vi "Pressure_cuff_3_tyler edit.vi"() -> ()   [LabVIEW 2016]
uses:
  <vilib>/Utility/miscctls.llb/LVBoundsTypeDef.ctl
  <vilib>/Instr/_visa.llb/VISA Configure Serial Port (Instr).vi
  <vilib>/Utility/file.llb/Write To Spreadsheet File (DBL).vi
  <vilib>/ptbypt/NI_PtbyPt.lvlib
panel:
  in  "?":enum32{"Serial Commands", "Operation"}(tab)
  in  "?":string="Instructions:\n\n1) Adjust Serial Commands appropriately using the \"Serial Commands\" tab and following the associated instructions.\n\nNote: There are two modes built into this system. The most basic mode is the \"Manual\" mode in which the continually defines the desired pressure throughout the experiment. The second mode is the \"Automatic\" mode in which the user can obtain a stair-step response by increasing/decreasing the pressure by user-defined increments of pressure every user-defined length of time.\n\n*When the \"Sync Auto/Manual\" indicator is illuminated, the program will maintain the same pressure when the user switches back and forth between the Manual and Automatic modes. This is the default setting."
  in  "Set Pump Mode":string="MOD PMP\r\n"
  in  "Set Diameter":string="11.001"
  in  "Set Direction to Refill":string="DIR REF\r\n"
  in  "Run1":string="RUN\r\n"
  in  "Stop":string="STP\r\n"
  in  "Set Fast Infusion Rate":string="1.0600"
  in  "Run":string="RUN\r\n"
  in  "Run4":string="RUN\r\n"
  in  "Set Direction to Infuse 2":string="DIR INF\r\n"
  in  "Run2":string="RUN\r\n"
  in  "Set Slow Infusion Rate":string="250.02"
  in  "Set Direction to Refill 2":string="DIR REF\r\n"
  in  "Run3":string="RUN\r\n"
  in  "Set Slow to Refill Rate":string="250.05"
  in  "Set Fast Refill Rate":string="1.0003"
  in  "Set Direction to Infuse":string="DIR INF\r\n"
  in  "D1":string="DIA "
  in  "D3":string="\r\n"
  in  "Set FRR":string="RFR "
  in  "Set FRR1":string=" MM\r\n"
  in  "Set FIR":string="RAT "
  in  "Set FIR1":string=" MM\r\n"
  in  "Set SIR":string="RAT "
  in  "Set SIR1":string=" UM\r\n"
  in  "Set SRR":string="RFR "
  in  "Set SRR1":string=" UM\r\n"
  in  "Set Initial Refill Rt":string="RFR 4.0003 MM\r\n"
  in  "Set Initial Infusion Rt":string="RAT 4.0600 MM\r\n"
  in  "r":dbl=7.0
  in  "baud rate 2":u32=9600
  in  "VISA resource name 2":refnum<visa-resource-name>="COM1"
  in  "data bits 2":u16=8 min=5 max=8 step=1
  in  "parity 2":u16(ring) items=["None", "Odd", "Even", "Mark", "Space"]
  in  "stop bits":u16(ring)=20 items=["1.0"=10, "1.5"=15, "2.0"=20]
  in  "flow control 2":u16(ring) items=["None"=0, "XON/XOFF"=1, "RTS/CTS"=2, "DTR/DSR"=4]
  in  "Automatic\nDeflate     Inflate 2":bool
  out "?":dbl(slide)=-0.9000220331410755
  in  "Sync Auto/Manual":bool=TRUE
  out "?":dbl=-0.9000220331410755 format="%#_3g"
  in  "Desired Pressure (mmHg)\n         (user defined)":dbl
  out "Measured Pressure (mmHg)":dbl=-0.9000220331410755
  in  "?":bool
  in  "?":bool=TRUE
  out "INFLATING":bool
  out "DEFLATING":bool
  in  "Filter?":bool=TRUE
  out "?":dbl(knob)=-0.9000220331410755 scale=0.0..80.0 scale format="%#_3g"
  out "Pressure vs. Time":cluster{"Y":dbl[], "Y":dbl[]}[](graph)=[{"Y"=[0.0, 0.10000991821289062, 0.20001983642578125, 0.3000297546386719, 0.4000396728515625, 0.5000495910644531, 0.600059986114502, 0.7000699043273926, 0.8000798225402832, 0.9000897407531738, 1.0000996589660645, 1.1001100540161133, 1.200119972229004, 1.3001298904418945, 1.4001398086547852, 1.5001497268676758, 1.6001596450805664, 1.7001700401306152, 1.8001799583435059, 1.9001898765563965, 2.000199794769287, 2.1002097129821777, 2.2002196311950684, 2.300230026245117, 2.400239944458008, 2.5002498626708984, 2.600259780883789, 2.7002696990966797, 2.8002796173095703, 2.900290012359619, 3.0002999305725098, 3.1003098487854004, 3.200319766998291, 3.3003296852111816, 3.4003396034240723], "Y"=[-0.13551515208114814, -0.5177685926111119, -0.26293296559113327, -0.42220523247861885, -0.4413179045051191, -0.5177685926111135, -0.5942192807171078, -0.8235713450350877, -0.8235713450350877, -0.8235713450350877, -0.9764727212470732, -0.8235713450350877, -0.9000220331410821, -0.9000220331410821, -1.0529234093530675, -1.2822754736710473, -1.664528914201013, -1.5880782260950184, -1.5880782260950184, -1.5880782260950184, -1.435176849883033, -1.0529234093530675, -0.9764727212470765, -1.0529234093530708, -1.1293740974590654, -1.2822754736710507, -1.5116275379890305, -1.664528914201016, -1.664528914201016, -1.8174302904130015, -1.5880782260950217, -1.3587261617770419, -1.3587261617770419, -1.2058247855650566, -0.9000220331410823]}, {"Y"=[0.0, 0.10000991821289062, 0.20001983642578125, 0.3000297546386719, 0.4000396728515625, 0.5000495910644531, 0.600059986114502, 0.7000699043273926, 0.8000798225402832, 0.9000897407531738, 1.0000996589660645, 1.1001100540161133, 1.200119972229004, 1.3001298904418945, 1.4001398086547852, 1.5001497268676758, 1.6001596450805664, 1.7001700401306152, 1.8001799583435059, 1.9001898765563965, 2.000199794769287, 2.1002097129821777, 2.2002196311950684, 2.300230026245117, 2.400239944458008, 2.5002498626708984, 2.600259780883789, 2.7002696990966797, 2.8002796173095703, 2.900290012359619, 3.0002999305725098, 3.1003098487854004, 3.200319766998291, 3.3003296852111816, 3.4003396034240723], "Y"=[0.0, 0.0, 0.0, 0.0, 0.0, 0.0, 0.0, 0.0, 0.0, 0.0, 0.0, 0.0, 0.0, 0.0, 0.0, 0.0, 0.0, 0.0, 0.0, 0.0, 0.0, 0.0, 0.0, 0.0, 0.0, 0.0, 0.0, 0.0, 0.0, 0.0, 0.0, 0.0, 0.0, 0.0, 0.0]}]
  out "Voltage In:":dbl=0.5150003631248783 format="%#_4g"
  out "Total Elapsed Time (s):":dbl=3.4003396034240723 format="%#_4g"
  in  "Which computer?":bool=TRUE
  in  "Automatic\nDeflate     Inflate":bool
  in  "Automatic      Manual":bool=TRUE
  in  "Automatic Starting\n       Pressure":dbl
  in  "?":string="Instructions:\n\n1) Adjust Serial Commands appropriately using the \"Serial Commands\" tab and following the associated instructions.\n\nNote: There are two modes built into this system. The most basic mode is the \"Manual\" mode in which the continually defines the desired pressure throughout the experiment. The second mode is the \"Automatic\" mode in which the user can obtain a stair-step response by increasing/decreasing the pressure by user-defined increments of pressure every user-defined length of time.\n\n*When the \"Sync Auto/Manual\" indicator is illuminated, the program will maintain the same pressure when the user switches back and forth between the Manual and Automatic modes. This is the default setting."
  out "Auto Desired":dbl=-80.0
  in  "Hold Time (s)\n     Desired":dbl=60.0
  out "Elapsed Time (s)\nsince P reached":dbl=3.4003396034240723 caption="Elapsed Time (s)"
  in  "Increment\n   (mmHg)":dbl=2.5
  # "- DO NOT CHANGE -\n  -  ANY OF THESE  -"
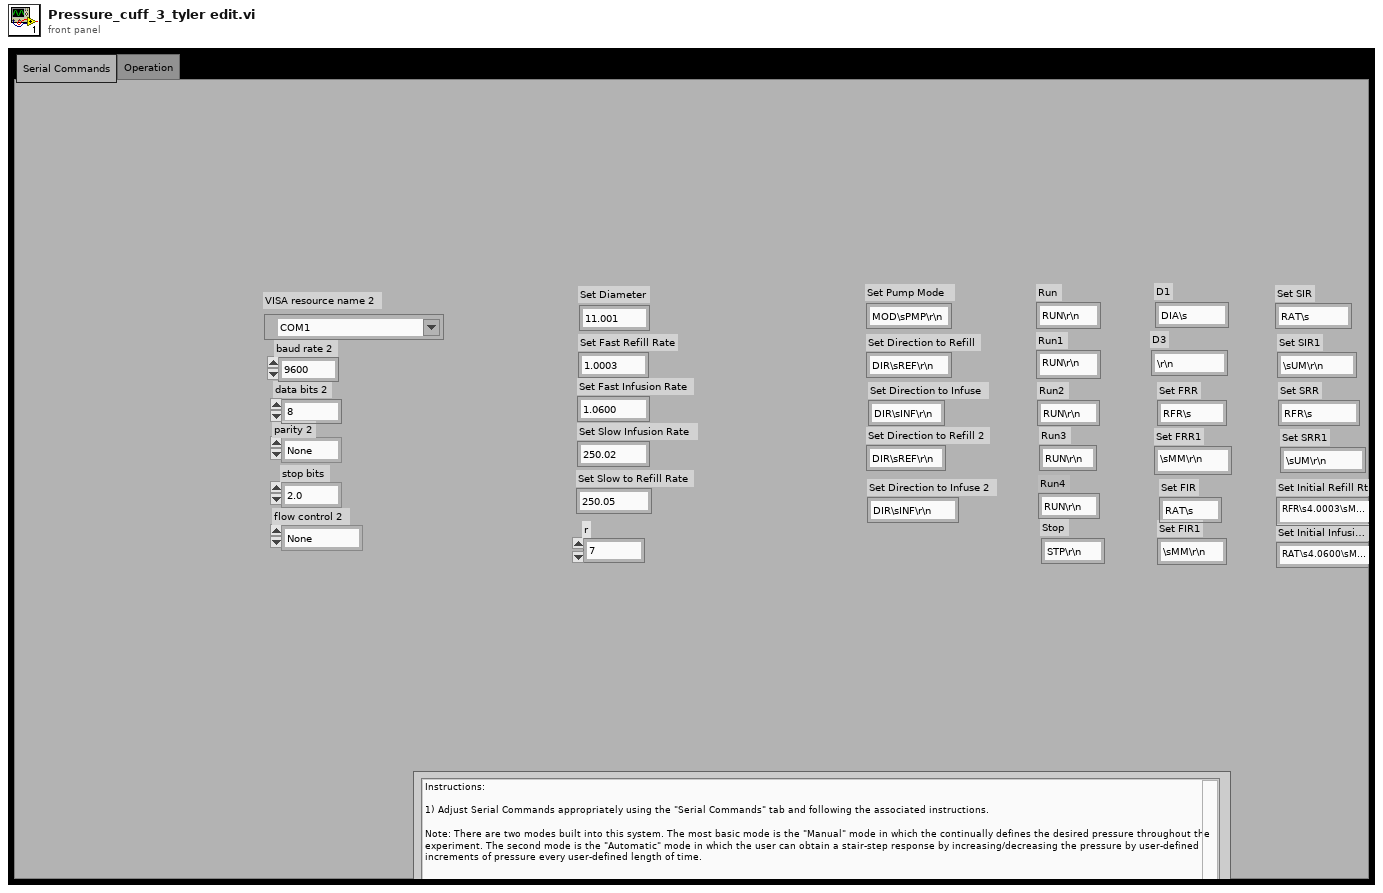
[diagram p1: front panel]
types:
  T1 = typedef "LVBoundsTypeDef.ctl" = cluster{"Width":u32, "Height":u32}
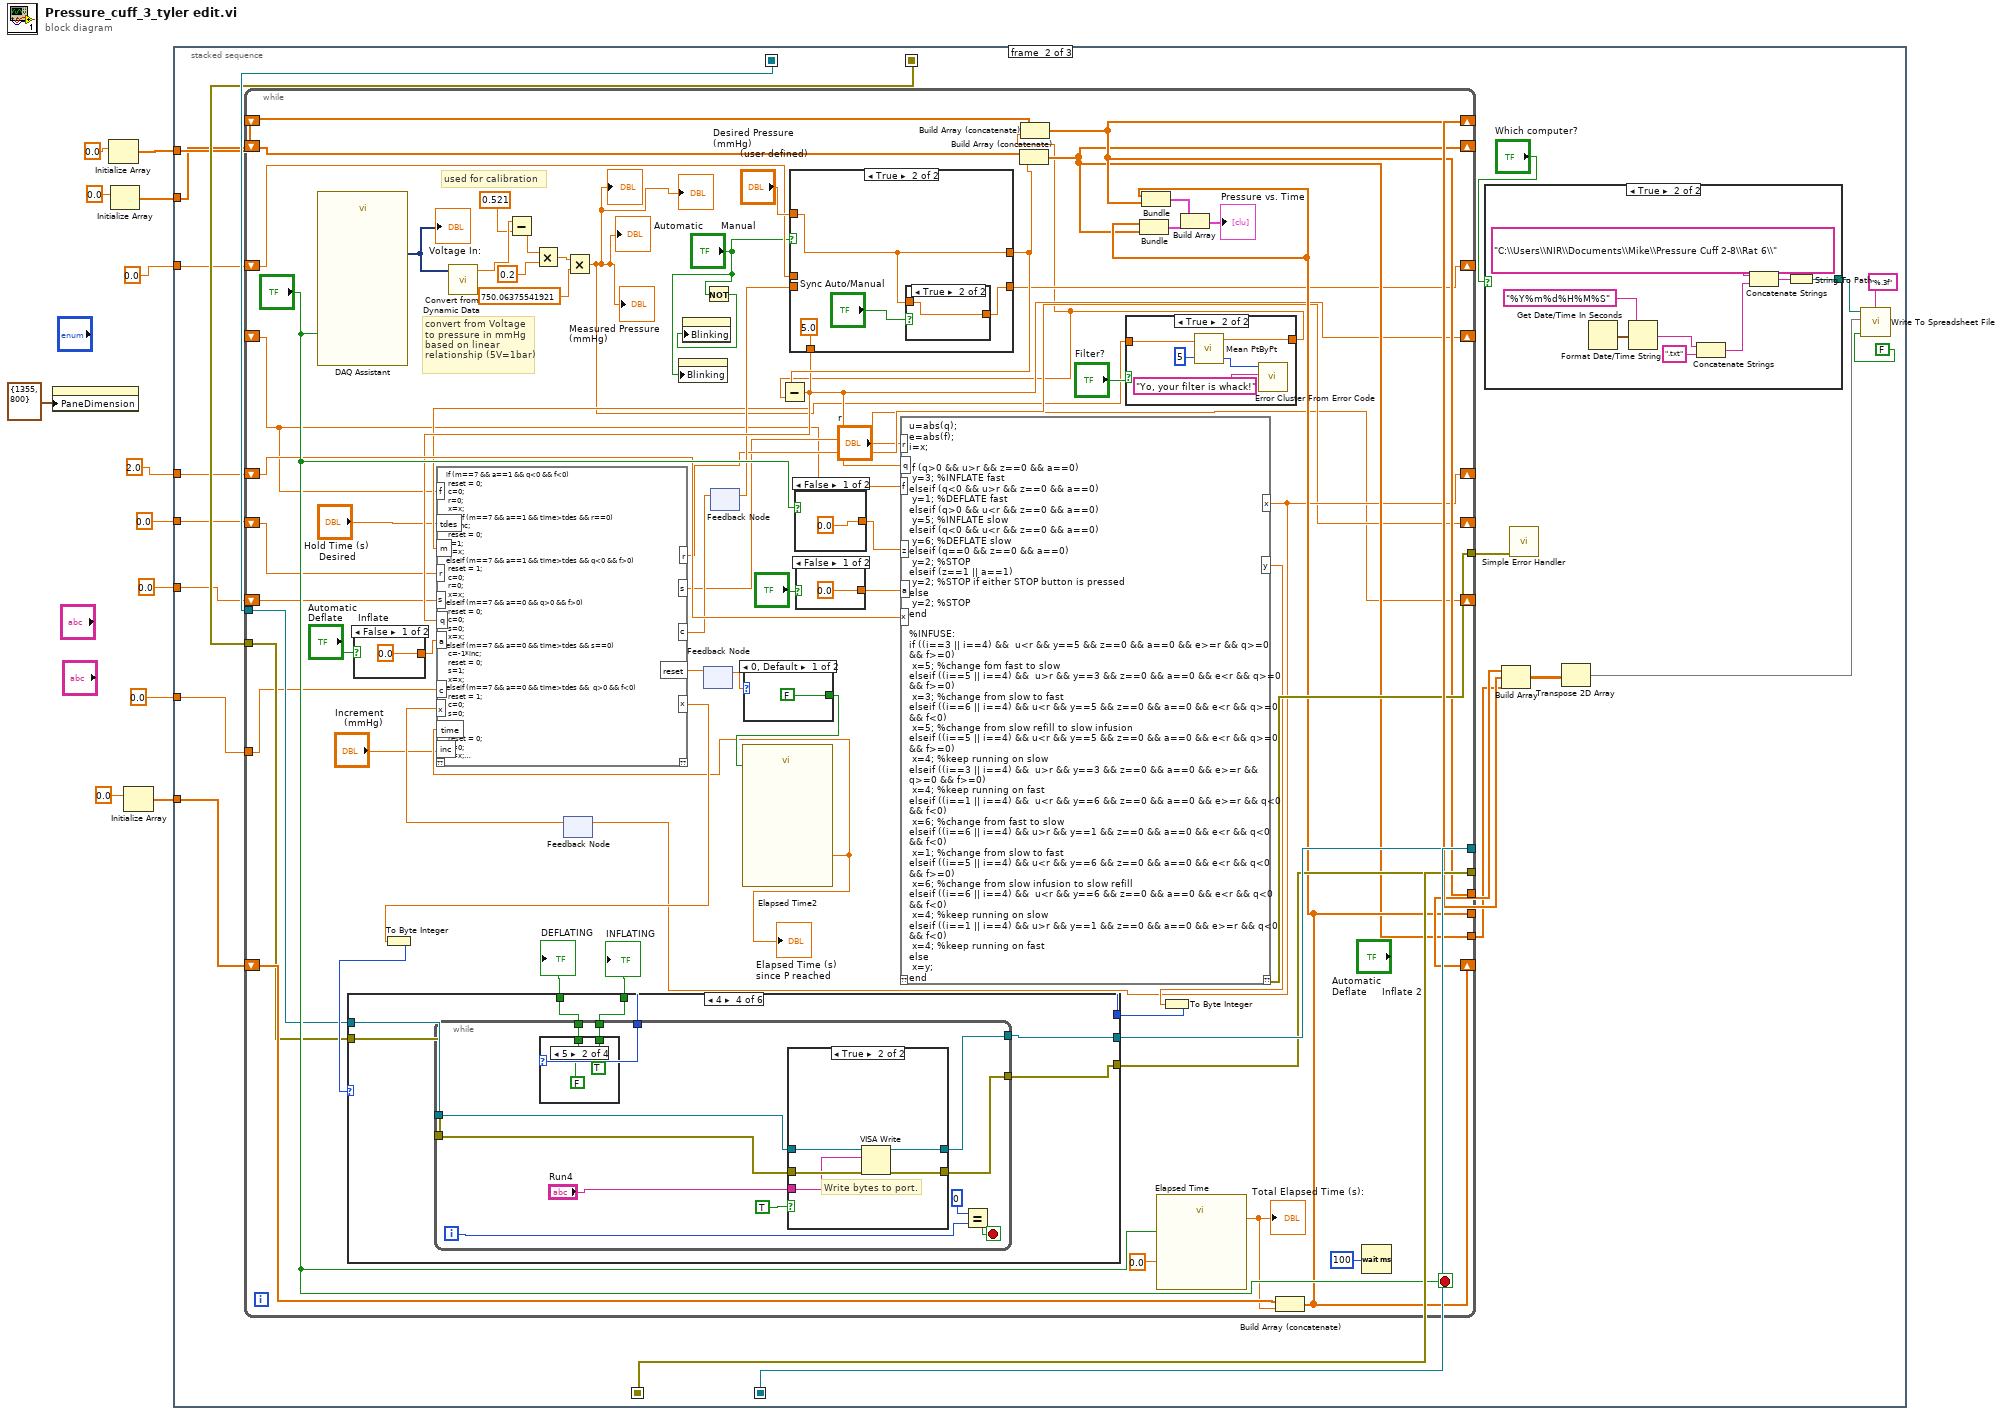
[diagram p0: block diagram]
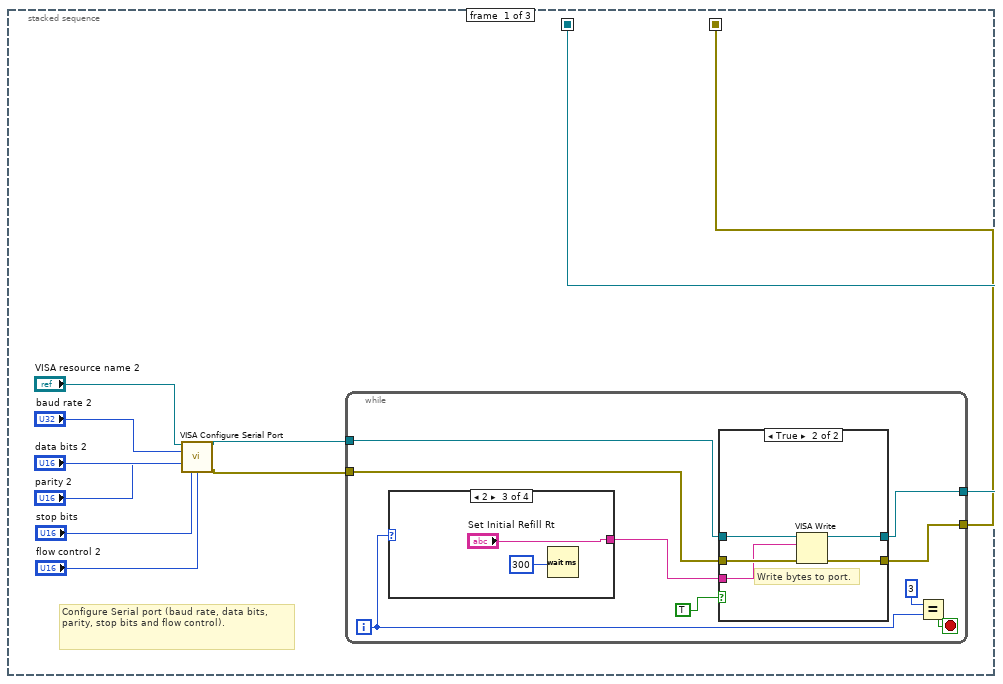
[diagram p2: hidden frame]
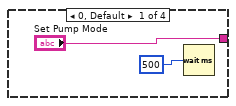
[diagram p3: hidden frame]
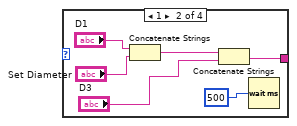
[diagram p4: hidden frame]
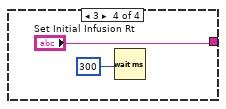
[diagram p5: hidden frame]
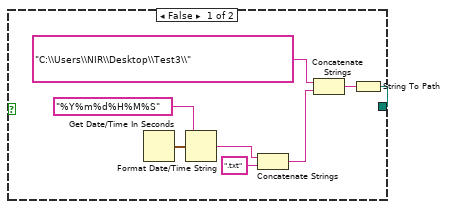
[diagram p7: hidden frame]
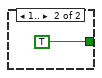
[diagram p8: hidden frame]
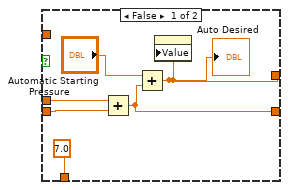
[diagram p9: hidden frame]
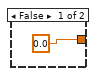
[diagram p10: hidden frame]
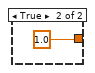
[diagram p11: hidden frame]
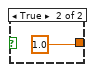
[diagram p13: hidden frame]
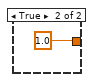
[diagram p14: hidden frame]
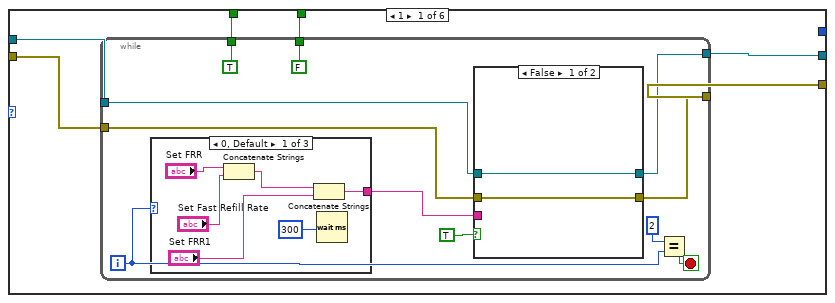
[diagram p15: hidden frame]
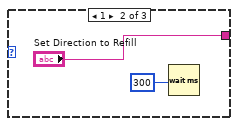
[diagram p16: hidden frame]
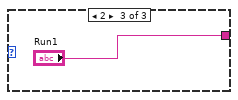
[diagram p17: hidden frame]
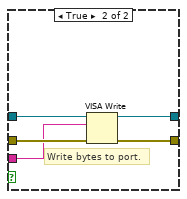
[diagram p18: hidden frame]
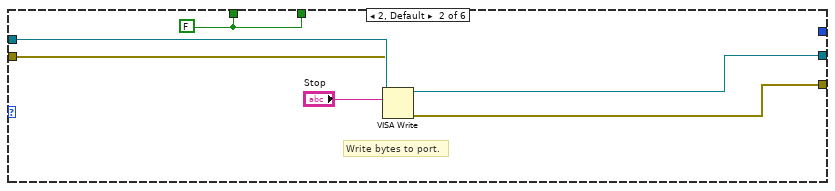
[diagram p19: hidden frame]
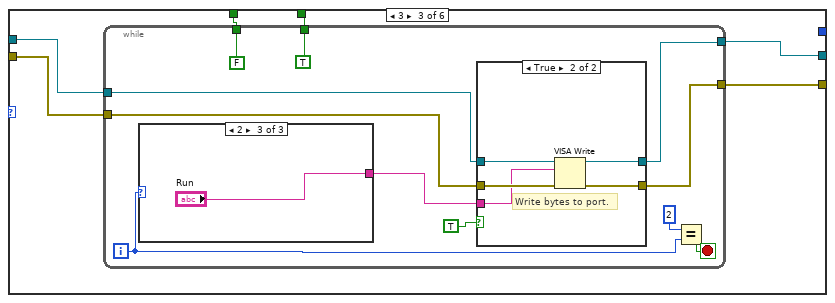
[diagram p20: hidden frame]
diagram:
  n1 = property class="TabCtl (strict)"("PaneDimension"=T1 {"Width"=1355, "Height"=800} ("Tab Control Pane Dimension")) -> ()  [unwired: 2 in, 2 out]
  n2 = Initialize Array(0.0 ("element")) -> (w12:dbl[])  [unwired: 1 in]
  n3 = Initialize Array(0.0 ("element")) -> (w9:dbl[])  [unwired: 1 in]
  n4 = Initialize Array(0.0 ("element")) -> (w7:dbl[])  [unwired: 1 in]
  n5 = stacked-sequence {
    seq-local: [w22 _ _] -> [_ w72 _]
    seq-local: [w21 _ _] -> [_ w71 _]
    seq-local: [_ w70 _] -> [_ _ w353]
    seq-local: [_ w69 _] -> [_ _ w351]
    tunnel: w12 -> [_ w59 _]
    tunnel: w9 -> [_ w58 _]
    tunnel: w7 -> [_ w57 _]
    tunnel: 0.0 ("input variable") -> [_ w55 _]
    tunnel: 0.0 -> [_ w54 _]
    tunnel: 0.0 -> [_ w53 _]
    tunnel: 2.0 -> [_ w52 _]
    tunnel: 0.0 ("element") -> [_ w51 _]
    frame #0 {
      # "Configure Serial port (baud rate, data bits, parity, stop bits and flow control)."
      n6 = call-poly "VISA Configure Serial Port"("VISA resource name"="VISA resource name 2", "baud rate (9600)"="baud rate 2", "data bits (8)"="data bits 2", "parity (0:none)"="parity 2", "stop bits (10: 1 bit)"="stop bits", "flow control (0:none)"="flow control 2") -> ("VISA resource name out"=w13:refnum<visa-resource-name>, "error out"=w14:errorcluster)  [unwired: 3 in, 5 out]
      n7 = while {
        tunnel: w13 -> [w31]
        tunnel: w14 -> [w30]
        tunnel: [w29] -> w22
        tunnel: [w28] -> w21
        i -> [w25]
        stop <- w24 stop-if-true
        n8 = case shown="2" w25 {
          tunnel: ["Set Pump Mode" w35 "Set Initial Refill Rt" "Set Initial Infusion Rt"] -> w27
          frame 0, Default {
            n9 = Wait (ms)(milliseconds to wait=u32 500) -> ()  [unwired: 1 out]
          }
          frame 1 {
            n10 = Concatenate Strings("D1", "Set Diameter") -> (w36:string)
            n11 = Concatenate Strings(w36, "D3") -> (w35:string)
            n12 = Wait (ms)(milliseconds to wait=u32 500) -> ()  [unwired: 1 out]
          }
          frame 2 {
            n13 = Wait (ms)(milliseconds to wait=u32 300) -> ()  [unwired: 1 out]
          }
          frame 3 {
            n14 = Wait (ms)(milliseconds to wait=u32 300) -> ()  [unwired: 1 out]
          }
        }
        n15 = case shown="True" TRUE ("write 1\nSet Up") {
          tunnel: [w45 w50] -> w28
          tunnel: w31 -> [w44 w49]
          tunnel: w30 -> [w45 w48]
          tunnel: [w44 w47] -> w29
          tunnel: w27 -> [_ w46]
          frame False {
          }
          frame True {
            # "Write bytes to port."
            n16 = VISA Write(VISA resource name=w49, write buffer=w46, error in (no error)=w48) -> (VISA resource name out=w47:refnum<visa-resource-name>, error out=w50:errorcluster)  [unwired: 1 out]
          }
        }
        n17 = Equal?(x=3, y=w25) -> (x = y?=w24:bool)
      }
    }
    frame #1 {
      n18 = while {
        shift-right: [w123] -> w61
        shift-left: w59 -> [w148]
        tunnel: [w123] -> _
        shift-right: [w127] -> w60
        shift-left: w57 -> [w149]
        tunnel: [w127] -> _
        tunnel: w71 -> [w140]
        tunnel: [w147] -> w70
        tunnel: [w146] -> w69
        tunnel: [w145] -> w62
        tunnel: w72 -> [w141]
        shift-right: [w114] -> _
        shift-left: w52 -> [w133]
        shift-right: [w117] -> _
        shift-left: _ -> [w103]
        shift-right: [w119] -> _
        shift-left: w58 -> [w132]
        tunnel: [w119] -> w56
        shift-right: [w111] -> _
        shift-left: w51 -> [w93]
        tunnel: w55 -> [w110]
        shift-right: [w107] -> _
        shift-left: w54 -> [w106]
        shift-right: [w105] -> _
        shift-left: w53 -> [w97]
        stop <- "?" stop-if-true
        # "used for calibration"
        # "convert from Voltage to pressure in mmHg\nbased on linear relationship (5V=1bar)"
        n19 = call "DAQ Assistant"("stop (T)"="?") -> ("data"=w125:dynamicdata)  [unwired: 16 in, 2 out]
        "Voltage In:" <- w125
        n20 = case shown="False" "Automatic\nDeflate     Inflate" {
          tunnel: [0.0 1.0] -> w116
          frame False {
          }
          frame True {
          }
        }
        n21 = call "Convert from Dynamic Data"("Dynamic Data Type"=w125) -> ("Scalar"=w122:dbl)  [unwired: 3 in]
        n22 = Subtract(x=w122, y=0.521) -> (x-y=w120:dbl)
        n23 = Multiply(x=w120, y=0.2) -> (x*y=w152:dbl)
        n24 = feedback #1() -> (w113:dbl)  [unwired: 1 in]
        n25 = Multiply(x=w152, y=750.06375541921) -> (x*y=w89:dbl)
        "Measured Pressure (mmHg)" <- w89
        "?" <- w89
        "?" <- w89
        "?" <- w89
        n26 = property on="Desired Pressure (mmHg)\n         (user defined)" class="DigNum (strict)"("Blinking"="Automatic      Manual") -> ()  [unwired: 2 in, 2 out]
        n27 = Not(x="Automatic      Manual") -> (.not. x?=w91:bool)
        n28 = property on="Auto Desired" class="DigNum (strict)"("Blinking"=w91) -> ()  [unwired: 2 in, 2 out]
        n29 = feedback #2() -> (w100:dbl)  [unwired: 1 in]
        n30 = feedback #3() -> (w108:dbl)  [unwired: 1 in]
        n31 = case shown="0, Default" w100 {
          tunnel: [FALSE TRUE] -> w102
          frame 0, Default {
          }
          frame 1.. {
          }
        }
        n32 = call "Elapsed Time2"("Reset"=w102) -> ("Elapsed Time (s)"=w98:dbl)  [unwired: 11 in, 7 out]
        "Elapsed Time (s)\nsince P reached" <- w98
        n33 = case shown="True" "Automatic      Manual" {
          tunnel: "Desired Pressure (mmHg)\n         (user defined)" -> [_ w163]
          tunnel: [w156 w163] -> w112
          tunnel: w108 -> [w161 _]
          tunnel: [w158 w162] -> w111
          tunnel: w93 -> [w159 _]
          tunnel: [7.0 5.0] -> w104
          frame False {
            n34 = Add(x=w159, y=w161) -> (x+y=w158:dbl)
            n35 = Add(x="Automatic Starting\n       Pressure", y=w158) -> (x+y=w156:dbl)
            "Auto Desired" <- w156
            n36 = property on="Desired Pressure (mmHg)\n         (user defined)" class="DigNum (strict)"("Value"=w156) -> ()  [unwired: 2 in, 2 out]
          }
          frame True {
            n37 = case shown="True" "Sync Auto/Manual" {
              tunnel: w163 -> [_ w167]
              tunnel: [0.0 w167] -> w162
              frame False {
              }
              frame True {
              }
            }
          }
        }
        n38 = case shown="False" "?" {
          tunnel: [0.0 1.0] -> w143
          frame False {
          }
          frame True {
          }
        }
        n39 = case shown="False" "?" {
          tunnel: [0.0 1.0] -> w138
          frame False {
          }
          frame True {
          }
        }
        n40 = Build Array (concatenate)(w132, w112) -> (w119:dbl[])
        n41 = case shown="True" "Filter?" {
          tunnel: w89 -> [w170 w174]
          tunnel: [w170 w173] -> w95
          frame False {
          }
          frame True {
            n42 = call <vilib>:"Mean PtByPt.vi"("x"=w174, "sample length"=5) -> ("mean"=w173:dbl, "error"=w171:i32)  [unwired: 2 in]
            n43 = call <vilib>:"Error Cluster From Error Code.vi"("error message (\"\")"="Yo, your filter is whack!" ("error message (\"\")"), "error code (0)"=w171) -> ()  [unwired: 7 in, 1 out]
          }
        }
        n44 = Subtract(x=w112, y=w95) -> (x-y=w117:dbl)
        n45 = script code="if (m==7 && a==1 && q<0 && f<0)\n reset = 0;\n c=0;\n r=0;\n x=x;\nelseif (m==7 && a==1 && time>tdes && r==0)\n c=inc;\n reset = 0;\n r=1;\n x=x;\nelseif (m==7 && a==1 && time>tdes && q<0 && f>0)\n reset = 1;\n c=0;\n r=0;\n x=x;\nelseif (m==7 && a==0 && q>0 && f>0)\n reset = 0;\n c=0;\n s=0;\n x=x;\nelseif (m==7 && a==0 && time>tdes && s==0)\n c=-1*inc;\n reset = 0;\n s=1;\n x=x;\nelseif (m==7 && a==0 && time>tdes &&  q>0 && f<0)\n reset = 1;\n c=0;\n s=0;\n x=x;\nelse\n reset = 0;\n c=0;\n x=x;\nend"("c"=w110, "x"=w113, "a"=w116, "q"=w117, "r"=w106, "s"=w97, "m"=w104, "f"=w103, "time"=w98, "tdes"="Hold Time (s)\n     Desired", "inc"="Increment\n   (mmHg)") -> ("c"=w109:dbl, "x"=w115:dbl, "r"=w107:dbl, "s"=w105:dbl, "reset"=w101:dbl)  [unwired: 1 in, 1 out]
        n46 = To Byte Integer(number=w115) -> (8bit integer=w144:i8)
        n47 = feedback-in #2(w101) -> ()
        n48 = feedback-in #3(w109) -> ()
        n49 = script code="u=abs(q);\ne=abs(f);\ni=x;\n\nif (q>0 && u>r && z==0 && a==0)\n y=3; %INFLATE fast\nelseif (q<0 && u>r && z==0 && a==0)\n y=1; %DEFLATE fast\nelseif (q>0 && u<r && z==0 && a==0)\n y=5; %INFLATE slow\nelseif (q<0 && u<r && z==0 && a==0)\n y=6; %DEFLATE slow\nelseif (q==0 && z==0 && a==0)\n y=2; %STOP\nelseif (z==1 || a==1)\n y=2; %STOP if either STOP button is pressed\nelse\n y=2; %STOP\nend\n\n%INFUSE:\nif ((i==3 || i==4) &&  u<r && y==5 && z==0 && a==0 && e>=r && q>=0 && f>=0)\n x=5; %change fom fast to slow\nelseif ((i==5 || i==4) &&  u>r && y==3 && z==0 && a==0 && e<r && q>=0 && f>=0)\n x=3; %change from slow to fast\nelseif ((i==6 || i==4) && u<r && y==5 && z==0 && a==0 && e<r && q>=0 && f<0)\n x=5; %change from slow refill to slow infusion\nelseif ((i==5 || i==4) && u<r && y==5 && z==0 && a==0 && e<r && q>=0 && f>=0)\n x=4; %keep running on slow\nelseif ((i==3 || i==4) &&  u>r && y==3 && z==0 && a==0 && e>=r && q>=0 && f>=0)\n x=4; %keep running on fast\nelseif ((i==1 || i==4) &&  u<r && y==6 && z==0 && a==0 && e>=r && q<0 && f<0)\n x=6; %change from fast to slow\nelseif ((i==6 || i==4) && u>r && y==1 && z==0 && a==0 && e<r && q<0 && f<0)\n x=1; %change from slow to fast\nelseif ((i==5 || i==4) && u<r && y==6 && z==0 && a==0 && e<r && q<0 && f>=0)\n x=6; %change from slow infusion to slow refill\nelseif ((i==6 || i==4) &&  u<r && y==6 && z==0 && a==0 && e<r && q<0 && f<0)\n x=4; %keep running on slow\nelseif ((i==1 || i==4) && u>r && y==1 && z==0 && a==0 && e>=r && q<0 && f<0)\n x=4; %keep running on fast\nelse\n x=y;\nend" ("Script Node")("z"=w143, "a"=w138, "x"=w133, "q"=w117, "f"=w103, "r"="r") -> ("??"=w145:errorcluster, "x"=w114:dbl, "y"=w135:dbl)  [unwired: 1 in]
        n50 = feedback-in #1(w114) -> ()
        n51 = Build Array (concatenate)(w148, w95) -> (w123:dbl[])
        n52 = call "Elapsed Time"("Auto Reset"="?", "Set Start Time (s)"=0.0) -> ("Elapsed Time (s)"=w131:dbl)  [unwired: 10 in, 7 out]
        "Total Elapsed Time (s):" <- w131
        n53 = To Byte Integer(number=w135) -> (8bit integer=w134:i8)
        n54 = case shown="4" w144 {
          tunnel: w141 -> [w183 w218 w224 w256 w289 w321]
          tunnel: w140 -> [w182 w217 w223 w255 w288 w320]
          tunnel: [w185 w216 w222 w258 w287 w319] -> w147
          tunnel: [w184 w215 w221 w257 w286 w318] -> w146
          tunnel: [w181 w213 w220 w252 w290 w323] -> w137
          tunnel: [w180 w213 w219 w253 w291 w322] -> w136
          tunnel: w134 -> [_ _ _ w254 _ _]
          frame 1 {
            n55 = while {
              tunnel: w183 -> [w196]
              tunnel: w182 -> [w195]
              tunnel: [w194] -> w185
              tunnel: [w193] -> w184
              tunnel: [TRUE ("DEFLATING")] -> w181
              tunnel: [FALSE] -> w180
              i -> [w190]
              stop <- w189 stop-if-true
              n56 = case shown="0, Default" w190 {
                tunnel: [w197 "Set Direction to Refill" "Run1"] -> w192
                frame 0, Default {
                  n57 = Concatenate Strings("Set FRR", "Set Fast Refill Rate") -> (w199:string)
                  n58 = Concatenate Strings(w199, "Set FRR1") -> (w197:string)
                  n59 = Wait (ms)(milliseconds to wait=u32 300) -> ()  [unwired: 1 out]
                }
                frame 1 {
                  n60 = Wait (ms)(milliseconds to wait=u32 300) -> ()  [unwired: 1 out]
                }
                frame 2 {
                }
              }
              n61 = case shown="False" TRUE {
                tunnel: [w207 w212] -> w193
                tunnel: w196 -> [w206 w211]
                tunnel: w195 -> [w207 w210]
                tunnel: [w206 w209] -> w194
                tunnel: w192 -> [_ w208]
                frame False {
                }
                frame True {
                  # "Write bytes to port."
                  n62 = VISA Write(VISA resource name=w211, write buffer=w208, error in (no error)=w210) -> (VISA resource name out=w209:refnum<visa-resource-name>, error out=w212:errorcluster)  [unwired: 1 out]
                }
              }
              n63 = Equal?(x=2, y=w190) -> (x = y?=w189:bool)
            }
          }
          frame 2, Default {
            w213 = FALSE
            # "Write bytes to port."
            n64 = VISA Write(VISA resource name=w218, write buffer="Stop", error in (no error)=w217) -> (VISA resource name out=w216:refnum<visa-resource-name>, error out=w215:errorcluster)  [unwired: 1 out]
          }
          frame 3 {
            n65 = while {
              tunnel: w224 -> [w235]
              tunnel: w223 -> [w234]
              tunnel: [w233] -> w222
              tunnel: [w232] -> w221
              tunnel: [FALSE] -> w220
              tunnel: [TRUE ("INFLATING")] -> w219
              i -> [w229]
              stop <- w228 stop-if-true
              n66 = case shown="2" w229 {
                tunnel: [w236 "Set Direction to Infuse" "Run"] -> w231
                frame 0, Default {
                  n67 = Concatenate Strings("Set FIR", "Set Fast Infusion Rate") -> (w238:string)
                  n68 = Concatenate Strings(w238, "Set FIR1") -> (w236:string)
                  n69 = Wait (ms)(milliseconds to wait=u32 300) -> ()  [unwired: 1 out]
                }
                frame 1 {
                  n70 = Wait (ms)(milliseconds to wait=u32 300) -> ()  [unwired: 1 out]
                }
                frame 2 {
                }
              }
              n71 = case shown="True" TRUE {
                tunnel: [w246 w251] -> w232
                tunnel: w235 -> [w245 w250]
                tunnel: w234 -> [w246 w249]
                tunnel: [w245 w248] -> w233
                tunnel: w231 -> [_ w247]
                frame False {
                }
                frame True {
                  # "Write bytes to port."
                  n72 = VISA Write(VISA resource name=w250, write buffer=w247, error in (no error)=w249) -> (VISA resource name out=w248:refnum<visa-resource-name>, error out=w251:errorcluster)  [unwired: 1 out]
                }
              }
              n73 = Equal?(x=2, y=w229) -> (x = y?=w228:bool)
            }
          }
          frame 4 {
            n74 = while {
              tunnel: w256 -> [w270]
              tunnel: w255 -> [w269]
              tunnel: [w268] -> w258
              tunnel: [w267] -> w257
              tunnel: w254 -> [w261]
              tunnel: [w260] -> w253
              tunnel: [w259] -> w252
              i -> [w262]
              stop <- w264 stop-if-true
              n75 = case shown="5" w261 {
                tunnel: [TRUE ("DEFLATING") TRUE ("DEFLATING") FALSE FALSE] -> w260
                tunnel: [FALSE FALSE TRUE ("DEFLATING") TRUE ("DEFLATING")] -> w259
                frame 3 {
                }
                frame 5 {
                }
                frame 6 {
                }
                frame 1, Default {
                }
              }
              n76 = case shown="True" TRUE {
                tunnel: [w280 w285] -> w267
                tunnel: w270 -> [w279 w284]
                tunnel: w269 -> [w280 w283]
                tunnel: [w279 w282] -> w268
                tunnel: "Run4" -> [_ w281]
                frame False {
                }
                frame True {
                  # "Write bytes to port."
                  n77 = VISA Write(VISA resource name=w284, write buffer=w281, error in (no error)=w283) -> (VISA resource name out=w282:refnum<visa-resource-name>, error out=w285:errorcluster)  [unwired: 1 out]
                }
              }
              n78 = Equal?(x=0, y=w262) -> (x = y?=w264:bool)
            }
          }
          frame 5 {
            n79 = while {
              tunnel: w289 -> [w301]
              tunnel: w288 -> [w300]
              tunnel: [w299] -> w287
              tunnel: [w298] -> w286
              tunnel: [FALSE] -> w290
              tunnel: [w292] -> w291
              i -> [w295]
              stop <- w294 stop-if-true
              w292 = TRUE
              n80 = case shown="0, Default" w295 {
                tunnel: [w302 "Set Direction to Infuse 2" "Run2"] -> w297
                frame 0, Default {
                  n81 = Concatenate Strings("Set SIR", "Set Slow Infusion Rate") -> (w304:string)
                  n82 = Wait (ms)(milliseconds to wait=u32 300) -> ()  [unwired: 1 out]
                  n83 = Concatenate Strings(w304, "Set SIR1") -> (w302:string)
                }
                frame 1 {
                  n84 = Wait (ms)(milliseconds to wait=u32 300) -> ()  [unwired: 1 out]
                }
                frame 2 {
                }
              }
              n85 = case shown="True" w292 {
                tunnel: [w312 w317] -> w298
                tunnel: w301 -> [w311 w316]
                tunnel: w300 -> [w312 w315]
                tunnel: [w311 w314] -> w299
                tunnel: w297 -> [_ w313]
                frame False {
                }
                frame True {
                  # "Write bytes to port."
                  n86 = VISA Write(VISA resource name=w316, write buffer=w313, error in (no error)=w315) -> (VISA resource name out=w314:refnum<visa-resource-name>, error out=w317:errorcluster)  [unwired: 1 out]
                }
              }
              n87 = Equal?(x=2, y=w295) -> (x = y?=w294:bool)
            }
          }
          frame 6 {
            n88 = while {
              tunnel: w321 -> [w334]
              tunnel: w320 -> [w333]
              tunnel: [w332] -> w319
              tunnel: [w331] -> w318
              tunnel: [TRUE ("DEFLATING")] -> w323
              tunnel: [FALSE] -> w322
              i -> [w328]
              stop <- w327 stop-if-true
              n89 = case shown="2" w328 {
                tunnel: [w336 "Set Direction to Refill 2" "Run3"] -> w330
                frame 0, Default {
                  n90 = Concatenate Strings("Set SRR", "Set Slow to Refill Rate") -> (w338:string)
                  n91 = Concatenate Strings(w338, "Set SRR1") -> (w336:string)
                  n92 = Wait (ms)(milliseconds to wait=u32 300) -> ()  [unwired: 1 out]
                }
                frame 1 {
                  n93 = Wait (ms)(milliseconds to wait=u32 300) -> ()  [unwired: 1 out]
                }
                frame 2 {
                }
              }
              n94 = case shown="True" TRUE {
                tunnel: [w345 w350] -> w331
                tunnel: w334 -> [w344 w349]
                tunnel: w333 -> [w345 w348]
                tunnel: [w344 w347] -> w332
                tunnel: w330 -> [_ w346]
                frame False {
                }
                frame True {
                  # "Write bytes to port."
                  n95 = VISA Write(VISA resource name=w349, write buffer=w346, error in (no error)=w348) -> (VISA resource name out=w347:refnum<visa-resource-name>, error out=w350:errorcluster)  [unwired: 1 out]
                }
              }
              n96 = Equal?(x=2, y=w328) -> (x = y?=w327:bool)
            }
          }
        }
        "DEFLATING" <- w137
        "INFLATING" <- w136
        n97 = Build Array (concatenate)(w149, w131) -> (w127:dbl[])
        n98 = Bundle(w127, w119) -> (w128:cluster{dbl[], dbl[]})  [unwired: 1 in]
        n99 = Bundle(w127, w123) -> (w129:cluster{dbl[], dbl[]})  [unwired: 1 in]
        n100 = Build Array(w129, w128) -> (→"Pressure vs. Time":cluster{dbl[], dbl[]}[])
        n101 = Wait (ms)(milliseconds to wait=u32 100) -> ()  [unwired: 1 out]
      }
      n102 = case shown="True" "Which computer?" {
        tunnel: [w73 w81] -> w68
        frame False {
          n103 = Get Date/Time In Seconds() -> (seconds since 1Jan1904=w80:timestamp)
          n104 = Format Date/Time String(time format string (%c)="%Y%m%d%H%M%S", seconds (now)=w80) -> (date/time string=w78:string)  [unwired: 1 in]
          n105 = Concatenate Strings(w78, ".txt" ("string")) -> (w75:string)
          n106 = Concatenate Strings("C:\\Users\\NIR\\Desktop\\Test3\\" ("Folder Path"), w75) -> (w74:string)
          n107 = String To Path(string=w74) -> (path=w73:path)
        }
        frame True {
          n108 = Get Date/Time In Seconds() -> (seconds since 1Jan1904=w88:timestamp)
          n109 = Format Date/Time String(time format string (%c)="%Y%m%d%H%M%S", seconds (now)=w88) -> (date/time string=w86:string)  [unwired: 1 in]
          n110 = Concatenate Strings(w86, ".txt" ("string")) -> (w83:string)
          n111 = Concatenate Strings("C:\\Users\\NIR\\Documents\\Mike\\Pressure Cuff 2-8\\Rat 6\\" ("Folder Path"), w83) -> (w82:string)
          n112 = String To Path(string=w82) -> (path=w81:path)
        }
      }
      n113 = Build Array(w60, w61, w56) -> (w65:dbl[][])
      n114 = call <vilib>:"Simple Error Handler.vi"("error in (no error)"=w62) -> ()  [unwired: 1 in, 8 out]
      n115 = Transpose 2D Array(2D array=w65) -> (transposed array=w64:dbl[][])
      n116 = call-poly <vilib>:"Write To Spreadsheet File.vi"("format (%.3f)"="%.3f", "append to file? (new file:F)"=FALSE, "2D data"=w64, "file path (dialog if empty)"=w68) -> ()  [unwired: 4 in, 1 out]
    }
    frame #2 {
      # "Note:Closing the serial port allows it to be used by other applications without quitting LabVIEW."
      # "Close session to port."
      n117 = VISA Close(VISA resource name=w353, error in (no error)=w351) -> (error out=w352:errorcluster)
      n118 = call <vilib>:"Simple Error Handler.vi"("error in (no error)"=w352) -> ()  [unwired: 1 in, 8 out]
    }
  }
